vi ".NET Type Builder Create Type.vi"(8 "error in (no error)":errorcluster, 9 ".NET Type Builder":refnum<k24>) -> (0 "error out":errorcluster, 1 ".NET Type":refnum<k24>)   [LabVIEW 2018, in "TwinCAT ADS.lvclass"]
uses:
  TwinCAT ADS.lvclass
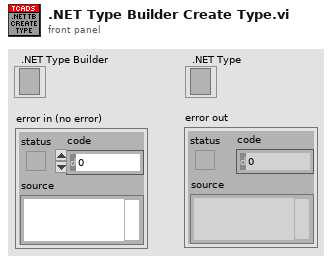
[diagram p1: front panel]
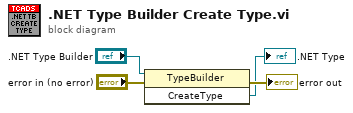
[diagram p0: block diagram]
diagram:
  n1 = invoke class="TypeBuilder" method="CreateType"(reference=".NET Type Builder", error in="error in (no error)") -> (error out=→"error out":errorcluster, "CreateType"=→".NET Type":refnum<k24>)  [unwired: 1 in, 1 out]
